vi "Create Level String.vi"(8 "Error In":errorcluster, 11 "Level":T1) -> (0 "Error Out":errorcluster, 3 "String":string)   [LabVIEW 2014, in "LV-Logger.lvlib"]
uses:
  LV-Logger.lvlib
  Public/Controls/Level.ctl
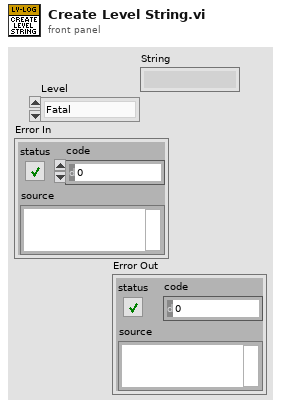
[diagram p1: front panel]
types:
  T1 = typedef "LV-Logger.lvlib/Level.ctl" = enum16{"Fatal", "Error", "Warn", "Info", "Debug", "Trace"}
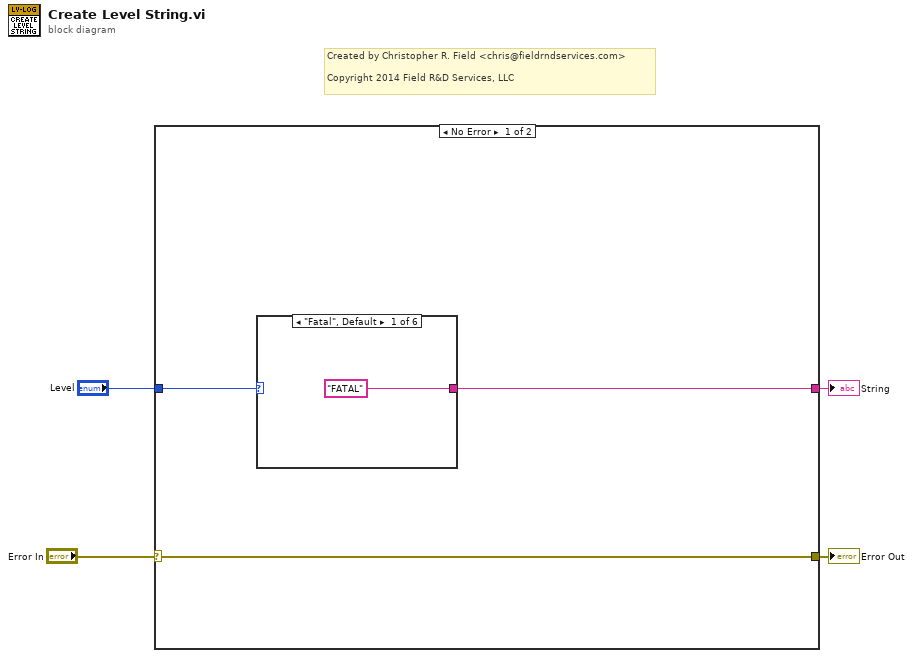
[diagram p0: block diagram]
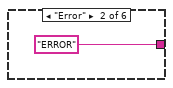
[diagram p2: hidden frame]
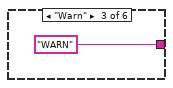
[diagram p3: hidden frame]
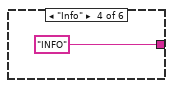
[diagram p4: hidden frame]
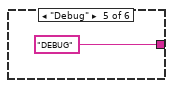
[diagram p5: hidden frame]
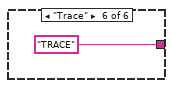
[diagram p6: hidden frame]
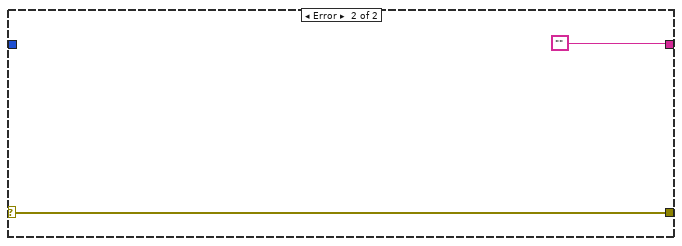
[diagram p7: hidden frame]
diagram:
  # "Created by Christopher R. Field <chris@fieldrndservices.com>\n\nCopyright 2014 Field R&D Services, LLC"
  n1 = case shown="No Error" "Error In" {
    selector: "Error In" -> [w5 w15]
    tunnel: "Level" -> [w7 _]
    tunnel: [w6 ""] -> w3
    tunnel: [w5 w15] -> w1
    frame No Error {
      n2 = case shown="\"Fatal\", Default" w7 {
        tunnel: ["FATAL" "ERROR" "WARN" "INFO" "DEBUG" "TRACE"] -> w6
        frame "Fatal", Default {
        }
        frame "Error" {
        }
        frame "Warn" {
        }
        frame "Info" {
        }
        frame "Debug" {
        }
        frame "Trace" {
        }
      }
    }
    frame Error {
    }
  }
  "String" <- w3
  "Error Out" <- w1
